vi "DSF Configuration from cluster.vi"(8 "error in (no error)":errorcluster, 11 "configuration cluster":T1) -> (0 "error out":errorcluster, 3 "DSFConfiguration out":refnum<class "DSFConfiguration.lvclass">)   [LabVIEW 2017, in "DSFConfiguration.lvclass"]
uses:
  DSFConfiguration.lvclass
  Controls/dsf configuration file/1.0.0/dsf timing.ctl
  Controls/dsf configuration file/1.0.0/dsf configuration file v1.0.0.lvlib
  Controls/dsf configuration file/1.0.0/dsf transfer.ctl
  Controls/dsf configuration file/1.0.0/dsf channel.ctl
  Controls/dsf configuration file/1.0.0/dsf settings.ctl
  Controls/dsf configuration file/1.0.0/dsf plugin.ctl
  Controls/dsf configuration file/1.0.0/dsf group.ctl
  Controls/dsf configuration file/1.0.0/dsf configuration.ctl
  Controls/dsf configuration file/1.0.0/version.ctl
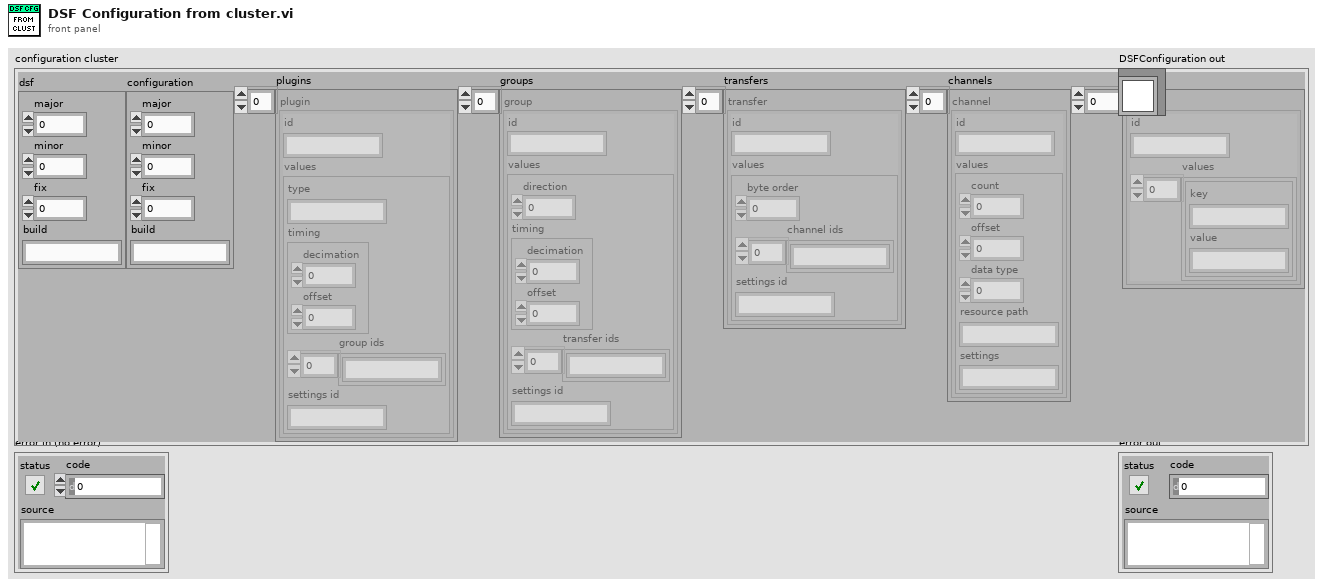
[diagram p1: front panel]
types:
  T1 = typedef "dsf configuration file v1.0.0.lvlib/dsf configuration.ctl" = cluster{"dsf":T2, "configuration":T2, "plugins":T3[], "groups":T5[], "transfers":T6[], "channels":T7[], "settings":T8[]}
  T2 = typedef "dsf configuration file v1.0.0.lvlib/version.ctl" = cluster{"major":u32, "minor":u32, "fix":u32, "build":string}
  T3 = typedef "dsf configuration file v1.0.0.lvlib/dsf plugin.ctl" = cluster{"id":string, "values":cluster{"type":string, "timing":T4, "group ids":string[], "settings id":string}}
  T4 = typedef "dsf configuration file v1.0.0.lvlib/dsf timing.ctl" = cluster{"decimation":i32, "offset":i32}
  T5 = typedef "dsf configuration file v1.0.0.lvlib/dsf group.ctl" = cluster{"id":string, "values":cluster{"direction":i32, "timing":T4, "transfer ids":string[], "settings id":string}}
  T6 = typedef "dsf configuration file v1.0.0.lvlib/dsf transfer.ctl" = cluster{"id":string, "values":cluster{"byte order":i32, "channel ids":string[], "settings id":string}}
  T7 = typedef "dsf configuration file v1.0.0.lvlib/dsf channel.ctl" = cluster{"id":string, "values":cluster{"count":i32, "offset":i32, "data type":dbl, "resource path":string, "settings":string}}
  T8 = typedef "dsf configuration file v1.0.0.lvlib/dsf settings.ctl" = cluster{"id":string, "values":cluster{"key":string, "value":string}[]}
  T9 = cluster{"count":i32, "offset":i32, "data type":dbl, "resource path":string, "settings":string}
  T10 = cluster{"byte order":i32, "channel ids":string[], "settings id":string}
  T11 = cluster{"direction":i32, "timing":T4, "transfer ids":string[], "settings id":string}
  T12 = cluster{"type":string, "timing":T4, "group ids":string[], "settings id":string}
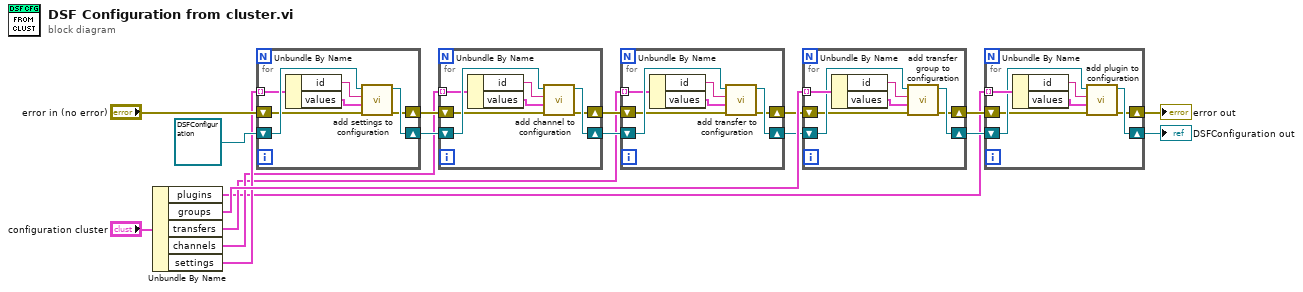
[diagram p0: block diagram]
diagram:
  n1 = Unbundle By Name("configuration cluster") -> ("plugins"=w3:T3[], "groups"=w11:T5[], "transfers"=w6:T6[], "channels"=w7:T7[], "settings"=w8:T8[])
  n2 = for {
    shift-right: [w24] -> w16
    shift-left: refnum<class "DSFConfiguration.lvclass"> refnum ("DSFConfiguration out") -> [w25]
    shift-right: [w20] -> w15
    shift-left: "error in (no error)" -> [w21]
    tunnel: w8 -> [w19] mode=indexing
    n3 = Unbundle By Name(w19) -> ("id"=w23:string, "values"=w22:cluster{"key":string, "value":string}[])
    n4 = call "add settings to configuration.vi"("error in (no error)"=w21, "user settings"=w22, "id"=w23, "DSFConfiguration in"=w25) -> ("error out"=w20:errorcluster, "DSFConfiguration out"=w24:refnum<class "DSFConfiguration.lvclass">)  [unwired: 6 in]
  }
  n5 = for {
    shift-right: [w31] -> w14
    shift-left: w16 -> [w32]
    shift-right: [w27] -> w13
    shift-left: w15 -> [w28]
    tunnel: w7 -> [w26] mode=indexing
    n6 = Unbundle By Name(w26) -> ("id"=w30:string, "values"=w29:T9)
    n7 = call "add channel to configuration.vi"("error in (no error)"=w28, "channel info"=w29, "id"=w30, "DSFConfiguration in"=w32) -> ("error out"=w27:errorcluster, "DSFConfiguration out"=w31:refnum<class "DSFConfiguration.lvclass">)  [unwired: 6 in]
  }
  n8 = for {
    shift-right: [w38] -> w10
    shift-left: w14 -> [w39]
    shift-right: [w34] -> w9
    shift-left: w13 -> [w35]
    tunnel: w6 -> [w33] mode=indexing
    n9 = Unbundle By Name(w33) -> ("id"=w37:string, "values"=w36:T10)
    n10 = call "add transfer to configuration.vi"("error in (no error)"=w35, "transfer info"=w36, "id"=w37, "DSFConfiguration in"=w39) -> ("error out"=w34:errorcluster, "DSFConfiguration out"=w38:refnum<class "DSFConfiguration.lvclass">)  [unwired: 6 in]
  }
  n11 = for {
    tunnel: w11 -> [w46] mode=indexing
    shift-right: [w44] -> w5
    shift-left: w10 -> [w45]
    shift-right: [w40] -> w4
    shift-left: w9 -> [w41]
    n12 = Unbundle By Name(w46) -> ("id"=w43:string, "values"=w42:T11)
    n13 = call "add transfer group to configuration.vi"("error in (no error)"=w41, "group info"=w42, "id"=w43, "DSFConfiguration in"=w45) -> ("error out"=w40:errorcluster, "DSFConfiguration out"=w44:refnum<class "DSFConfiguration.lvclass">)  [unwired: 6 in]
  }
  n14 = for {
    tunnel: w3 -> [w53] mode=indexing
    shift-right: [w51] -> w1
    shift-left: w5 -> [w52]
    shift-right: [w47] -> w2
    shift-left: w4 -> [w48]
    n15 = Unbundle By Name(w53) -> ("id"=w50:string, "values"=w49:T12)
    n16 = call "add plugin to configuration.vi"("error in (no error)"=w48, "plugin info"=w49, "id"=w50, "DSFConfiguration in"=w52) -> ("error out"=w47:errorcluster, "DSFConfiguration out"=w51:refnum<class "DSFConfiguration.lvclass">)  [unwired: 6 in]
  }
  "error out" <- w2
  "DSFConfiguration out" <- w1
